vi "MyG#G3SubTempl_Create.vi"(0 "reference in":refnum<class "MyG#G3SubTempl.lvclass">, 1 "MyAttribute":dbl, 2 "MySubAttribute":dbl, 5 "error in (no error)":errorcluster) -> (14 "reference out":refnum<class "MyG#G3SubTempl.lvclass">, 19 "error out":errorcluster)   [LabVIEW 2020, in "MyG#G3SubTempl.lvclass"]
doc: "Constructor."
uses:
  MyG#G3SubTempl.lvclass
  C:/ProjectGSharpDevelopment_2020-3/gsharp/VIPM/Files/vi.lib/addons/_AddQ/G#Object/G#Object.lvclass
  C:/ProjectGSharpDevelopment_2020-3/gsharp/VIPM/Files/examples/Object-Oriented G# Development/CreateDestroy/MyG#G3Templ_class/MyG#G3Templ.lvclass
  vi.lib/addons/_AddQ/G#Object/G#Object.lvclass
  MyG#G3Templ_class/MyG#G3Templ.lvclass
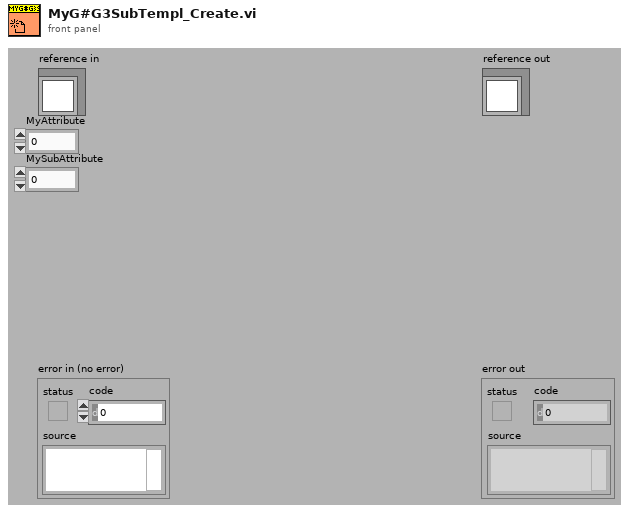
[diagram p1: front panel]
types:
  T1 = typedef "MyG#G3SubTempl.lvclass/ObjectAttributes.ctl" = cluster{"Base class":T2, "MySubAttribute":dbl}
  T2 = typedef "MyG#G3Templ.lvclass/ObjectAttributes.ctl" = cluster{"MyAttribute":dbl}
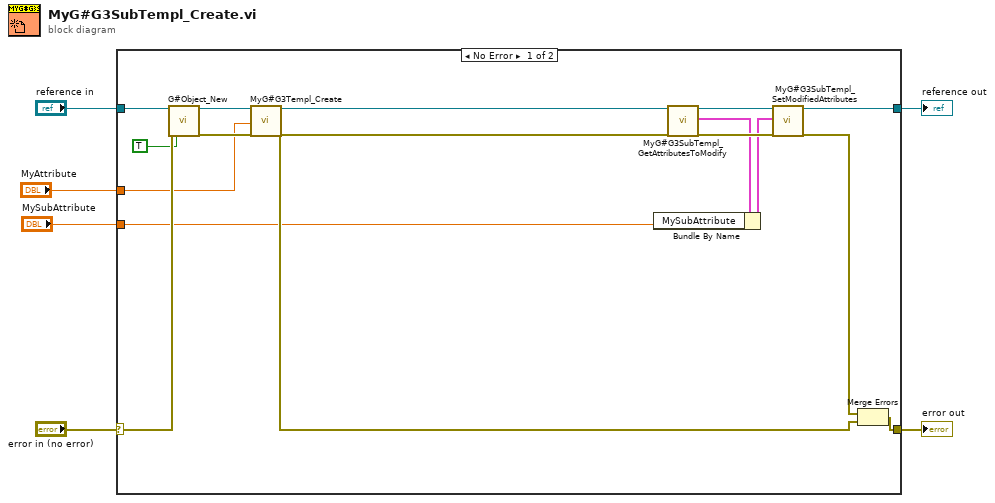
[diagram p0: block diagram]
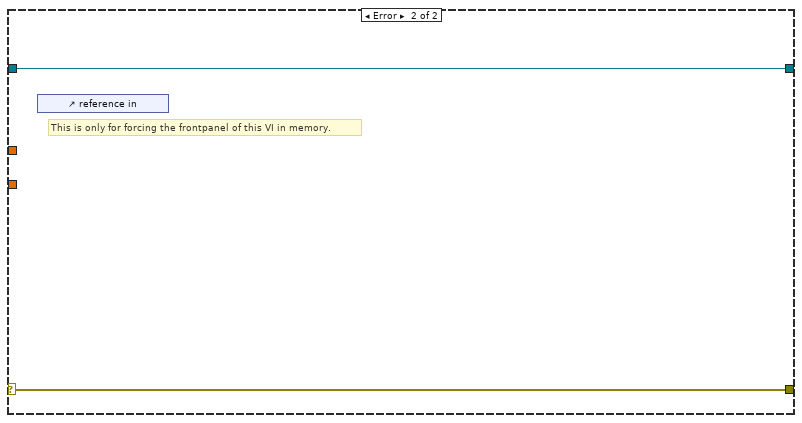
[diagram p2: hidden frame]
diagram:
  n1 = case shown="No Error" "error in (no error)" {
    selector: "error in (no error)" -> [w21 w24]
    tunnel: [w20 w24] -> w5
    tunnel: [w14 w23] -> w3
    tunnel: "reference in" -> [w22 w23]
    tunnel: "MyAttribute" -> [w8 _]
    tunnel: "MySubAttribute" -> [w7 _]
    frame No Error {
      n2 = call "G#Object_New.vi"("reference in"=w22, "error in (no error)"=w21, "user counter (T)?"=TRUE ("User Counter")) -> ("reference out"=w19:refnum<class "MyG#G3SubTempl.lvclass">, "error out"=w18:errorcluster)  [unwired: 14 in, 1 out]
      n3 = call "MyG#G3Templ_Create.vi"("reference in"=w19, "MyAttribute"=w8, "error in (no error)"=w18) -> ("reference out"=w15:refnum<class "MyG#G3SubTempl.lvclass">, "error out"=w13:errorcluster)  [unwired: 15 in]
      n4 = call "MyG#G3SubTempl_GetAttributesToModify.vi"("reference in"=w15, "error in (no error)"=w13) -> ("reference out"=w16:refnum<class "MyG#G3SubTempl.lvclass">, "attributes"=w10:T1, "error out"=w12:errorcluster)  [unwired: 13 in, 2 out]
      n5 = Bundle By Name(cluster=w10, "MySubAttribute"=w7) -> (w9:T1)
      n6 = call "MyG#G3SubTempl_SetModifiedAttributes.vi"("reference in"=w16, "attributes"=w9, "error in (no error)"=w12) -> ("reference out"=w14:refnum<class "MyG#G3SubTempl.lvclass">, "error out"=w11:errorcluster)  [unwired: 15 in]
      n7 = Merge Errors(w11, w13) -> (w20:errorcluster)
    }
    frame Error {
      # "This is only for forcing the frontpanel of this VI in memory."
      n8 = control-ref of="reference in"() -> ()  [unwired: 1 out]
    }
  }
  "error out" <- w5
  "reference out" <- w3
